vi "HeaterLoop.vi"(8 "Error In":errorcluster, 10 "Heater Data":refnum<notifier>, 11 "Action Queues":T1) -> (0 "Error Out":errorcluster)   [LabVIEW 2012]
uses:
  HeaterAction.ctl
  HeaterActionQueueElement.ctl
  UIAction.ctl
  UIActionQueueElement.ctl
  libs/Omega-CSi32/Omega-CSi32.lvlib
  <vilib>/Utility/error.llb/DialogType.ctl
  ActionQueues.ctl
  LogActionQueueElement.ctl
  LogAction.ctl
  HardwareActionQueueElement.ctl
  HardwareAction.ctl
  MFCAction.ctl
  MFCActionQueueElement.ctl
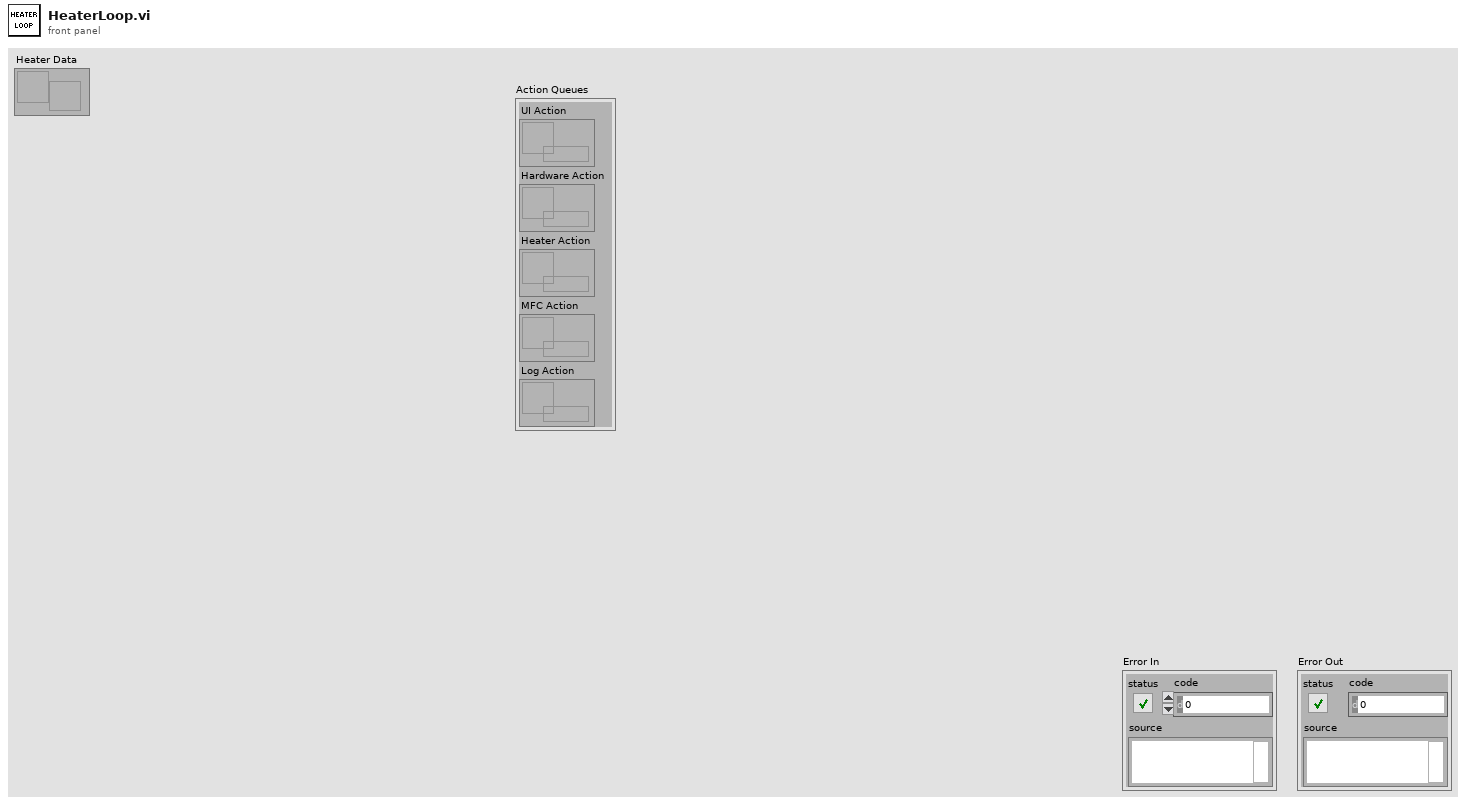
[diagram p1: front panel]
types:
  T1 = typedef "ActionQueues.ctl" = cluster{"UI Action":refnum<queue>, "Hardware Action":refnum<queue>, "Heater Action":refnum<queue>, "MFC Action":refnum<queue>, "Log Action":refnum<queue>}
  T2 = typedef "UIActionQueueElement.ctl" = cluster{"Action":T3, "Data":variant}
  T3 = typedef "UIAction.ctl" = enum16{"Initialize", "Connect", "MFC Connected", "Heater Connected", "Disconnect", "MFC Disconnected", "Heater Disconnected", "Configure MFC", "Configure Heater", "Open Log", "Close Log", "Shutdown"}
  T4 = typedef "HeaterActionQueueElement.ctl" = cluster{"Action":T5, "Data":variant}
  T5 = typedef "HeaterAction.ctl" = enum16{"Initialize", "Start", "Read", "Write", "Stop", "Error", "Shutdown"}
  T6 = typedef "DialogType.ctl" = u16
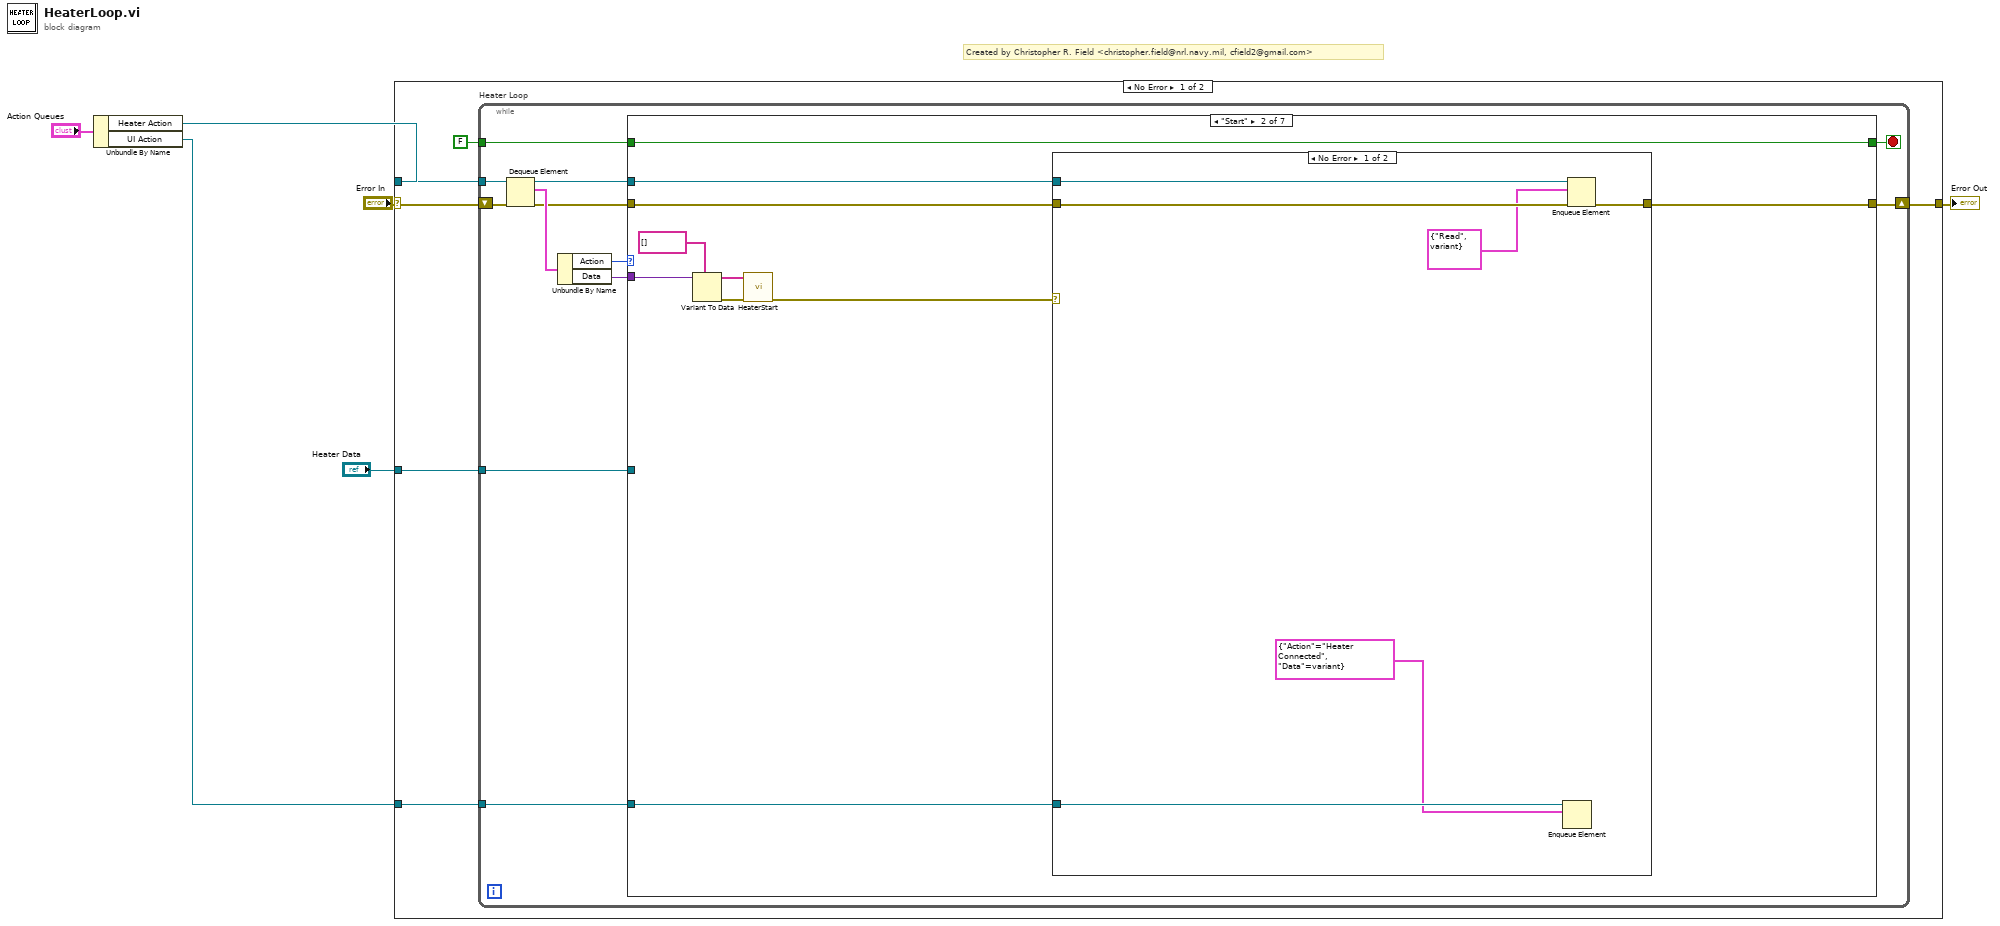
[diagram p0: block diagram]
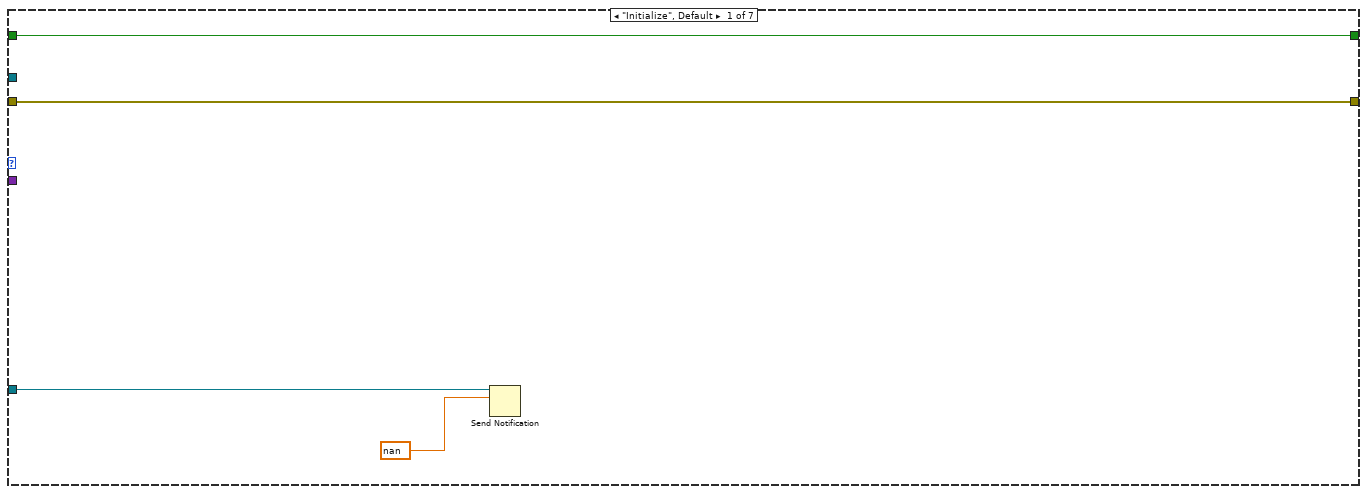
[diagram p2: hidden frame]
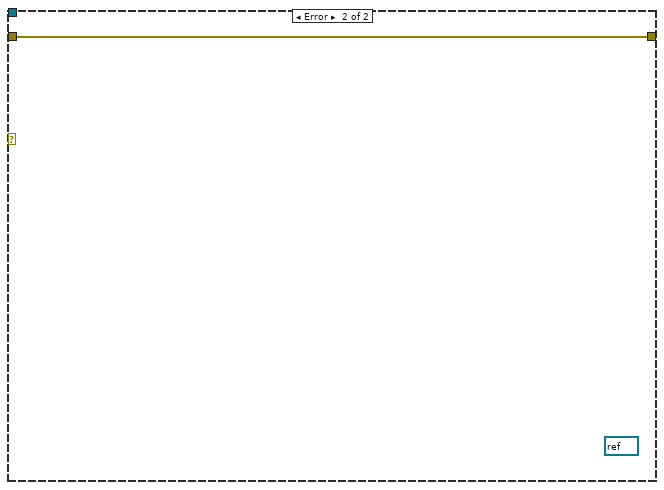
[diagram p3: hidden frame]
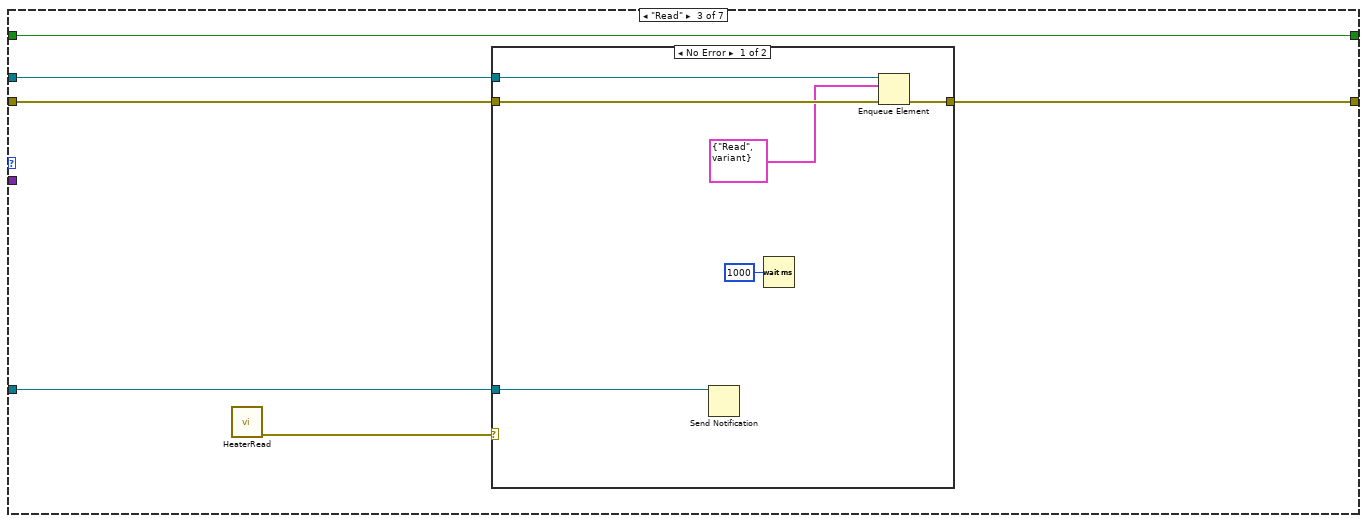
[diagram p4: hidden frame]
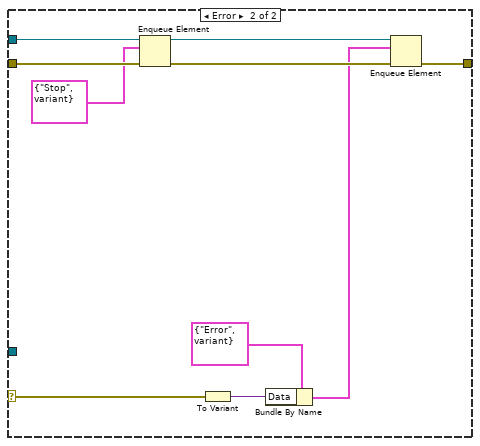
[diagram p5: hidden frame]
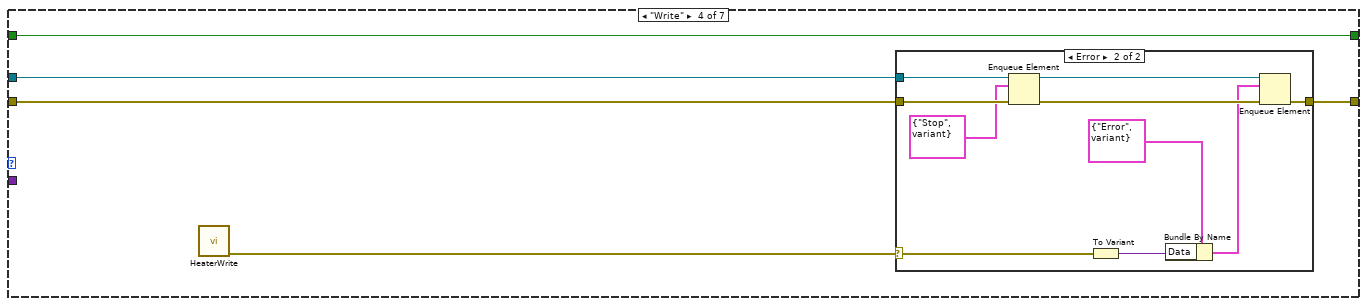
[diagram p6: hidden frame]
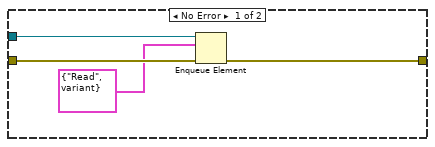
[diagram p7: hidden frame]
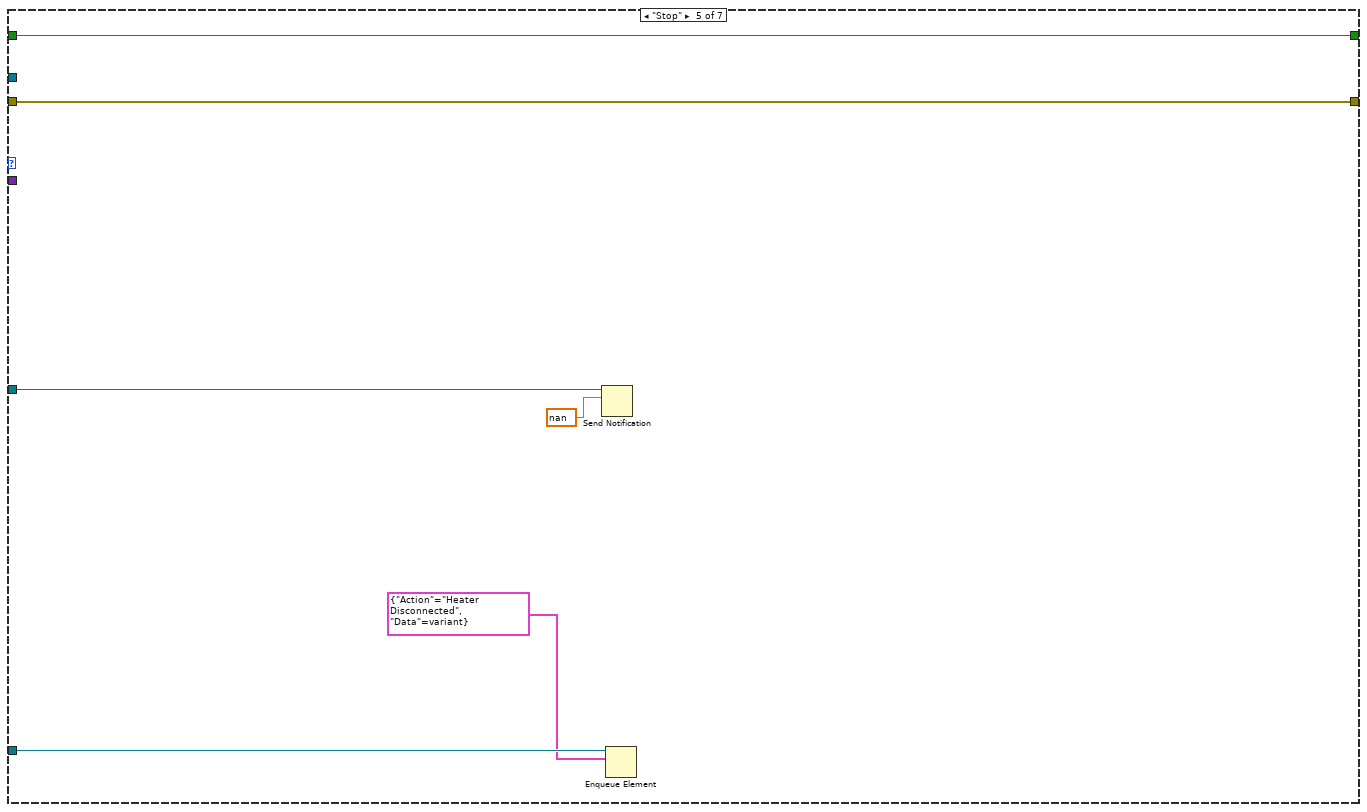
[diagram p8: hidden frame]
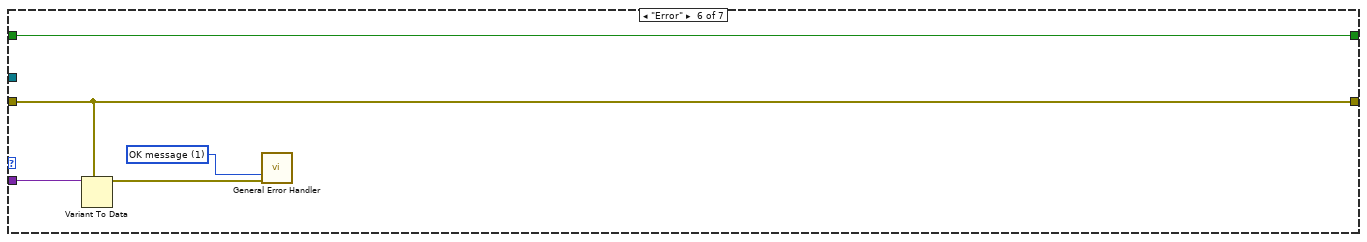
[diagram p9: hidden frame]
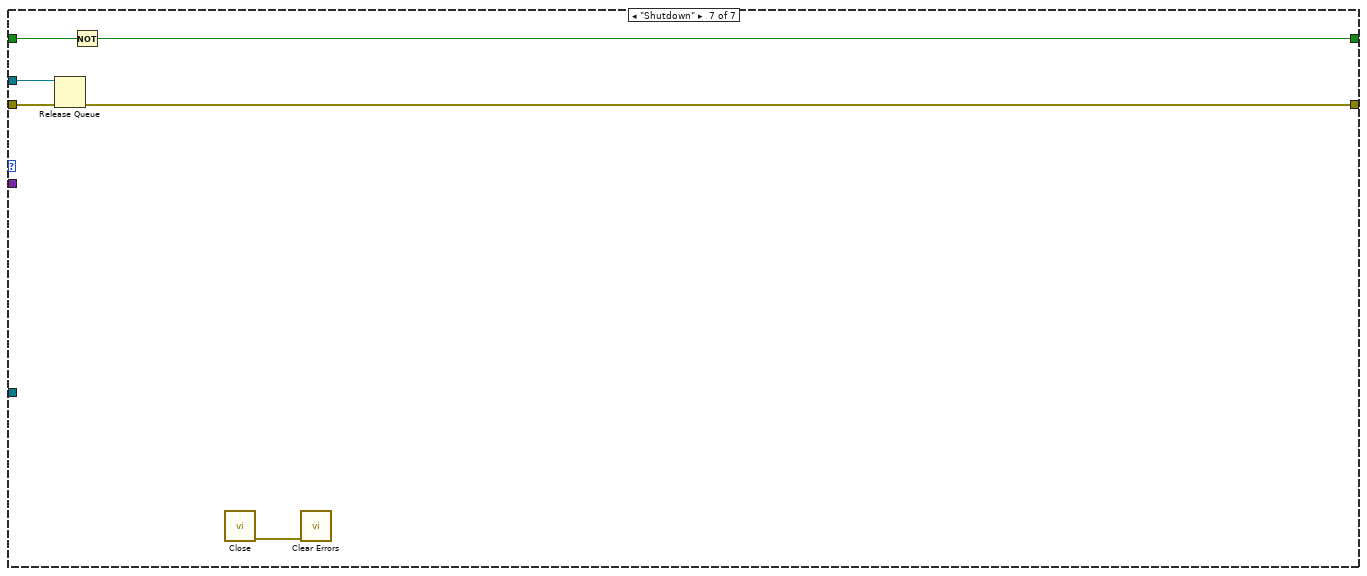
[diagram p10: hidden frame]
diagram:
  # "Created by Christopher R. Field <christopher.field@nrl.navy.mil, cfield2@gmail.com>"
  n1 = Unbundle By Name("Action Queues") -> ("Heater Action"=w3:refnum<queue>, "UI Action"=w2:refnum<queue>)
  n2 = case shown="No Error" "Error In" {
    selector: "Error In" -> [w11 w104]
    tunnel: w3 -> [w10 _]
    tunnel: [w9 w104] -> w5
    tunnel: w2 -> [w8 _]
    tunnel: "Heater Data" -> [w7 _]
    frame No Error {
      n3 = while "Heater Loop" {
        tunnel: FALSE -> [w24]
        shift-right: [w18] -> w9
        shift-left: w11 -> [w23]
        tunnel: w10 -> [w15]
        tunnel: w8 -> [w14]
        tunnel: w7 -> [w13]
        stop <- w16 stop-if-true
        n4 = Dequeue Element(queue=w15, error in (no error)=w23) -> (queue out=w17:refnum<queue>, element=w22:T4, error out=w19:errorcluster)  [unwired: 1 in, 1 out]
        n5 = Unbundle By Name(w22) -> ("Action"=w21:T5, "Data"=w20:variant)
        n6 = case shown="\"Start\"" w21 {
          tunnel: w24 -> [w27 w38 w51 w72 w92 w97 w103]
          tunnel: w20 -> [_ w33 _ _ _ w96 _]
          tunnel: w19 -> [w28 w36 w49 w70 w91 w95 w100]
          tunnel: [w28 w35 w48 w69 w91 w95 w99] -> w18
          tunnel: w17 -> [_ w37 w50 w71 _ _ w101]
          tunnel: [w27 w38 w51 w72 w92 w97 w102] -> w16
          tunnel: w14 -> [_ w34 _ _ w90 _ _]
          tunnel: w13 -> [w26 _ w46 _ w89 _ _]
          frame "Initialize", Default {
            n7 = Send Notification(notification=nan, notifier=w26) -> ()  [unwired: 1 in, 2 out]
          }
          frame "Start" {
            n8 = Variant To Data(type=string[] [] ("VISA Resource List"), Variant=w33) -> (data=w31:string[], error out=w30:errorcluster)  [unwired: 1 in]
            n9 = call "HeaterStart.vi"("Error In"=w30, "VISA Resource List"=w31) -> ("Error Out"=w29:errorcluster)  [unwired: 9 in]
            n10 = case shown="No Error" w29 {
              tunnel: w37 -> [w44 _]
              tunnel: w36 -> [w43 w45]
              tunnel: [w42 w45] -> w35
              tunnel: w34 -> [w40 _]
              frame No Error {
                n11 = Enqueue Element(queue=w40, element=T2 {"Action"=enum."Heater Connected", "Data"=variant}) -> ()  [unwired: 2 in, 3 out]
                n12 = Enqueue Element(queue=w44, element=T4 {"Action"=enum."Read", "Data"=variant}, error in (no error)=w43) -> (error out=w42:errorcluster)  [unwired: 1 in, 2 out]
              }
              frame Error {
                (unwired) refnum<visa-resource-name> refnum ("CSi32 Out")
              }
            }
          }
          frame "Read" {
            n13 = call "HeaterRead.vi"() -> ("Error Out"=w47:errorcluster)  [unwired: 11 in]
            n14 = case shown="No Error" w47 {
              selector: w47 -> [_ w64]
              tunnel: w50 -> [w57 w63]
              tunnel: w49 -> [w56 w62]
              tunnel: [w55 w67] -> w48
              tunnel: w46 -> [w53 _]
              frame No Error {
                n15 = Send Notification(notifier=w53) -> ()  [unwired: 2 in, 2 out]
                n16 = Wait (ms)(milliseconds to wait=u32 1000) -> ()  [unwired: 1 out]
                n17 = Enqueue Element(queue=w57, element=T4 {"Action"=enum."Read", "Data"=variant}, error in (no error)=w56) -> (error out=w55:errorcluster)  [unwired: 1 in, 2 out]
              }
              frame Error {
                n18 = Enqueue Element(queue=w63, element=T4 {"Action"=enum."Stop", "Data"=variant}, error in (no error)=w62) -> (queue out=w59:refnum<queue>, error out=w60:errorcluster)  [unwired: 1 in, 1 out]
                n19 = To Variant(anything=w64) -> (Variant=w65:variant)
                n20 = Bundle By Name(cluster=T4 {"Action"=enum."Error", "Data"=variant} ("element"), "Data"=w65) -> (w58:T4)
                n21 = Enqueue Element(queue=w59, element=w58, error in (no error)=w60) -> (error out=w67:errorcluster)  [unwired: 1 in, 2 out]
              }
            }
          }
          frame "Write" {
            n22 = call "HeaterWrite.vi"() -> ("Error Out"=w68:errorcluster)  [unwired: 10 in, 1 out]
            n23 = case shown="Error" w68 {
              selector: w68 -> [_ w78]
              tunnel: w71 -> [w76 w86]
              tunnel: w70 -> [w75 w85]
              tunnel: [w73 w81] -> w69
              frame No Error {
                n24 = Enqueue Element(queue=w76, element=T4 {"Action"=enum."Read", "Data"=variant}, error in (no error)=w75) -> (error out=w73:errorcluster)  [unwired: 1 in, 2 out]
              }
              frame Error {
                n25 = Enqueue Element(queue=w86, element=T4 {"Action"=enum."Stop", "Data"=variant}, error in (no error)=w85) -> (queue out=w83:refnum<queue>, error out=w82:errorcluster)  [unwired: 1 in, 1 out]
                n26 = To Variant(anything=w78) -> (Variant=w79:variant)
                n27 = Bundle By Name(cluster=T4 {"Action"=enum."Error", "Data"=variant} ("element"), "Data"=w79) -> (w77:T4)
                n28 = Enqueue Element(queue=w83, element=w77, error in (no error)=w82) -> (error out=w81:errorcluster)  [unwired: 1 in, 2 out]
              }
            }
          }
          frame "Stop" {
            n29 = Send Notification(notification=nan, notifier=w89) -> ()  [unwired: 1 in, 2 out]
            n30 = Enqueue Element(queue=w90, element=T2 {"Action"=enum."Heater Disconnected", "Data"=variant}) -> ()  [unwired: 2 in, 3 out]
          }
          frame "Error" {
            w93 = T6 1 items=["no dialog", "OK message", "continue or stop message", "OK message + warnings", "continue/stop + warnings"] ("type of dialog (OK msg:1)")
            n31 = Variant To Data(type=w95, Variant=w96) -> (data=w94:errorcluster)  [unwired: 1 in, 1 out]
            n32 = call <vilib>:"General Error Handler.vi"("type of dialog (OK msg:1)"=w93, "error in (no error)"=w94) -> ()  [unwired: 9 in, 5 out]
          }
          frame "Shutdown" {
            n33 = Release Queue(queue=w101, error in (no error)=w100) -> (error out=w99:errorcluster)  [unwired: 1 in, 2 out]
            n34 = Not(x=w103) -> (.not. x?=w102:bool)
            n35 = call "Close.vi"() -> ("Error Out"=w98:errorcluster)  [unwired: 11 in]
            n36 = call <vilib>:"Clear Errors.vi"("error in (no error)"=w98) -> ()  [unwired: 6 in, 1 out]
          }
        }
      }
    }
    frame Error {
    }
  }
  "Error Out" <- w5
